vi "PicohrdlClose.vi"(8 "error in (no error)":errorcluster, 11 "Handle in":i16=16384) -> (0 "error out":errorcluster, 3 "handle":i16)   [LabVIEW 2010]
doc: "Calls HRDLCloseUnit()"
uses:
  PicoHRDL.dll
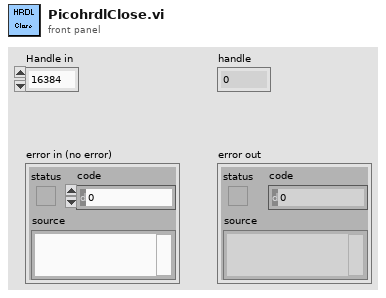
[diagram p1: front panel]
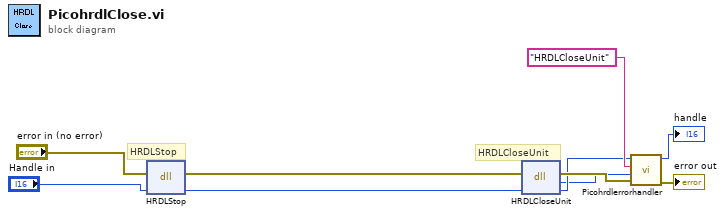
[diagram p0: block diagram]
diagram:
  # "HRDLStop"
  # "HRDLCloseUnit"
  n1 = dll-call lib="picohrdl.dll" fn="HRDLStop"(error in="error in (no error)", "handle"="Handle in") -> (error out=w1:errorcluster, "handle"=w2:i16)  [unwired: 3 in, 1 out]
  n2 = dll-call lib="PicoHRDL.dll" fn="HRDLCloseUnit"(error in=w1, "handle"=w2) -> (error out=w5:errorcluster, "return type"=w3:i16, "handle"=w4:i16)  [unwired: 2 in, 1 out]
  n3 = call "Picohrdlerrorhandler.vi"("Handle in"=w4, "API function"="HRDLCloseUnit", "Return"=w3, "error in (no error)"=w5) -> ("Handle out"=→"handle":i16, "error out"=→"error out":errorcluster)  [unwired: 5 in]
